vi "Time of Day.vi"() -> (3 "current time":timestamp format="%<%I:%M:%S %p\n%x>T")   [LabVIEW 2010]
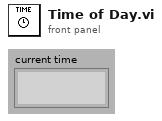
[diagram p1: front panel]
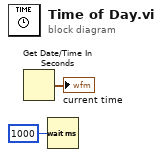
[diagram p0: block diagram]
diagram:
  n1 = Get Date/Time In Seconds() -> (seconds since 1Jan1904=→"current time":timestamp)
  n2 = Wait (ms)(milliseconds to wait=u32 1000) -> ()  [unwired: 1 out]
